vi "FT10_Fornax Mono1 Coag Power Down.vi"(11 "Message Handling Cluster in":T1={"Fornax Connected?"=refnum, "Unitherm Connected?"=refnum, "M4X Connected?"=refnum, "Unitherm Connect/Disconnect"=refnum, "Fornax Connection"=refnum, "UNITHERM Connection"="", "M4X Connection"=0, "FPGA VI Reference Out"=refnum, "PXI-7854R Connected?"=refnum, "Fornax Connect/Disconnect"=refnum, "7854 Connect/Disconnect"=refnum, "M4X Connect/Disconnect"=refnum, "Config cluster"={"Unitherm Port"="", "Simulate Values"=FALSE, "Fornax Connect Attempts"=0}, "Log Queue"=refnum, "Log Analysis Cluster - Current"={"RMS"=0.0, "Envelope Frequency"=0.0, "Peak"=0.0, "Crest Factor"=0.0, "Duty Cyle %"=0.0, "P-P"=0.0, "Frequency"=0.0, "THD"=0.0, "Postive Peak"=0.0, "Negative Peak"=0.0, "Mag_H1"=0.0, "Phase_H1"=0.0, "Mag_H3"=0.0, "Phase_H3"=0.0, "Mag_H5"=0.0, "Phase_H5"=0.0}, "Log Waveform Cluster - Current"={"t0"=timestamp(0 s since 1904-01-01), "dt"=1.0, "Y"=[]}, "Log Time"=timestamp(0 s since 1904-01-01), "Log Flag"=FALSE, "Log - Activation Settings Cluster"={"Log - Unitherm Load"="", "Log - Port"="", "Log - Mode"="", "Log - Power Level"=""}, "Log - Port Mode Cluster"={"Mono1 Cut Enum"=enum."Pure", "Mono2 Cut Enum"=enum."Pure", "Mono1 Coag Enum"=enum."Fulgerate", "Mono2 Coag Enum"=enum."Fulgerate", "Bipolar Enum"=enum."Standard"}, "Log Analysis Cluster - Diff Voltage"={"RMS"=0.0, "Envelope Frequency"=0.0, "Peak"=0.0, "Crest Factor"=0.0, "Duty Cyle %"=0.0, "P-P"=0.0, "Frequency"=0.0, "THD"=0.0, "Postive Peak"=0.0, "Negative Peak"=0.0, "Mag_H1"=0.0, "Phase_H1"=0.0, "Mag_H3"=0.0, "Phase_H3"=0.0, "Mag_H5"=0.0, "Phase_H5"=0.0}, "Log Waveform Cluster - Diff Voltage"={"t0"=timestamp(0 s since 1904-01-01), "dt"=1.0, "Y"=[]}, "Indicator Cluster"={"Mono1 - Cut Power"=refnum, "Mono1 - Coag Power"=refnum, "Mono2 - Cut Power"=refnum, "Mono2 - Coag Power"=refnum, "Bipolar Power"=refnum, "Mono1 Cut Enum"=refnum, "Mono1 Coag Enum"=refnum, "Mono2 Cut Enum"=refnum, "Mono2 Coag Enum"=refnum, "Bipolar Enum"=refnum}, "Log Power Level Cluster"={"Log Mono1 Cut Power"="", "Log Mono1 Coag Power"="", "Log Mono2 Cut Power"="", "Log Mono2 Coag Power"="", "Log Bipolar Power"=""}, "Footswitch Cluster"={"PXI-2565 reset device (boolean value)"=TRUE, "topology name"="2565/16-SPST", "PXI-2565 simulate (boolean value)"=FALSE, "PXI-2565 resource name"=""}}) -> (3 "Message Handling Cluster out":T1={"Fornax Connected?"=refnum, "Unitherm Connected?"=refnum, "M4X Connected?"=refnum, "Unitherm Connect/Disconnect"=refnum, "Fornax Connection"=refnum, "UNITHERM Connection"="", "M4X Connection"=0, "FPGA VI Reference Out"=refnum, "PXI-7854R Connected?"=refnum, "Fornax Connect/Disconnect"=refnum, "7854 Connect/Disconnect"=refnum, "M4X Connect/Disconnect"=refnum, "Config cluster"={"Unitherm Port"="", "Simulate Values"=FALSE, "Fornax Connect Attempts"=0}, "Log Queue"=refnum, "Log Analysis Cluster - Current"={"RMS"=0.0, "Envelope Frequency"=0.0, "Peak"=0.0, "Crest Factor"=0.0, "Duty Cyle %"=0.0, "P-P"=0.0, "Frequency"=0.0, "THD"=0.0, "Postive Peak"=0.0, "Negative Peak"=0.0, "Mag_H1"=0.0, "Phase_H1"=0.0, "Mag_H3"=0.0, "Phase_H3"=0.0, "Mag_H5"=0.0, "Phase_H5"=0.0}, "Log Waveform Cluster - Current"={"t0"=timestamp(0 s since 1904-01-01), "dt"=1.0, "Y"=[]}, "Log Time"=timestamp(0 s since 1904-01-01), "Log Flag"=FALSE, "Log - Activation Settings Cluster"={"Log - Unitherm Load"="", "Log - Port"="", "Log - Mode"="", "Log - Power Level"=""}, "Log - Port Mode Cluster"={"Mono1 Cut Enum"=enum."Pure", "Mono2 Cut Enum"=enum."Pure", "Mono1 Coag Enum"=enum."Fulgerate", "Mono2 Coag Enum"=enum."Fulgerate", "Bipolar Enum"=enum."Standard"}, "Log Analysis Cluster - Diff Voltage"={"RMS"=0.0, "Envelope Frequency"=0.0, "Peak"=0.0, "Crest Factor"=0.0, "Duty Cyle %"=0.0, "P-P"=0.0, "Frequency"=0.0, "THD"=0.0, "Postive Peak"=0.0, "Negative Peak"=0.0, "Mag_H1"=0.0, "Phase_H1"=0.0, "Mag_H3"=0.0, "Phase_H3"=0.0, "Mag_H5"=0.0, "Phase_H5"=0.0}, "Log Waveform Cluster - Diff Voltage"={"t0"=timestamp(0 s since 1904-01-01), "dt"=1.0, "Y"=[]}, "Indicator Cluster"={"Mono1 - Cut Power"=refnum, "Mono1 - Coag Power"=refnum, "Mono2 - Cut Power"=refnum, "Mono2 - Coag Power"=refnum, "Bipolar Power"=refnum, "Mono1 Cut Enum"=refnum, "Mono1 Coag Enum"=refnum, "Mono2 Cut Enum"=refnum, "Mono2 Coag Enum"=refnum, "Bipolar Enum"=refnum}, "Log Power Level Cluster"={"Log Mono1 Cut Power"="", "Log Mono1 Coag Power"="", "Log Mono2 Cut Power"="", "Log Mono2 Coag Power"="", "Log Bipolar Power"=""}, "Footswitch Cluster"={"PXI-2565 reset device (boolean value)"=TRUE, "topology name"="2565/16-SPST", "PXI-2565 simulate (boolean value)"=FALSE, "PXI-2565 resource name"=""}})   [LabVIEW 2024]
doc: "Decrease power level on Mono1 Coag"
uses:
  Controls/Control_Message Handling Cluster.ctl
  Controls/Control_M4X Connection.ctl
  Controls/Control_PXI-7854R FPGA Reference.ctl
  Controls/Control_Config Cluster.ctl
  Controls/Control_Config Unitherm Port.ctl
  Controls/Control_Config Simulate Values.ctl
  Controls/Control_Config Fornax Connect Attempts.ctl
  Controls/Control_Log Queue.ctl
  Controls/Control_Log Cluster.ctl
  Controls/Control_Log Time.ctl
  Controls/Control_Log Waveform Cluster - Current.ctl
  Controls/Control_Log Analysis Cluster - Current.ctl
  Controls/Control_Log Activation Settings Cluster.ctl
  Controls/Control_Log Unitherm Load.ctl
  Controls/Control_Log Port.ctl
  Controls/Control_Log Mode.ctl
  Controls/Control_Log Power Level.ctl
  Controls/Control_Log Waveform Cluster - Diff Voltage.ctl
  Controls/Control_Log Analysis Cluster - Diff Voltage.ctl
  Controls/Control_Log Flag.ctl
  Controls/Control_Log Port Mode Cluster.ctl
  Controls/Control_Fornax Mono1 Cut Enum.ctl
  Controls/Control_Fornax Mono2 Cut Enum.ctl
  Controls/Control_Fornax Mono1 Coag Enum.ctl
  Controls/Control_Fornax Mono2 Coag Enum.ctl
  Controls/Control_Fornax Bipolar Enum.ctl
  Controls/Control_Indicator Cluster.ctl
  Controls/Control_Log Power Level Cluster.ctl
  Controls/Control_Log Mono1 Cut Power.ctl
  Controls/Control_Log Mono1 Coag Power.ctl
  Controls/Control_Log Mono2 Cut Power.ctl
  Controls/Control_Log Mono2 Coag Power.ctl
  Controls/Control_Log Bipolar Power.ctl
  Controls/Control_Footswitch Reset Device Bool.ctl
  <instrlib>/niSwitch/niSwitch.llb/niSwitch Topologies.ctl
  Controls/Control_Footswitch Simulate Bool.ctl
  Controls/Control_Footswitch Resource Name.ctl
  Controls/Control_Fornax Generator.ctl
  Controls/Control_Fornax Energy Channel ID.ctl
  Controls/Control_Fornax Instrument Type.ctl
  Controls/Control_Fornax Parameter Type.ctl
  Controls/Control_Fornax Parameter Value.ctl
  Controls/Control_Fornax Energy Mode.ctl
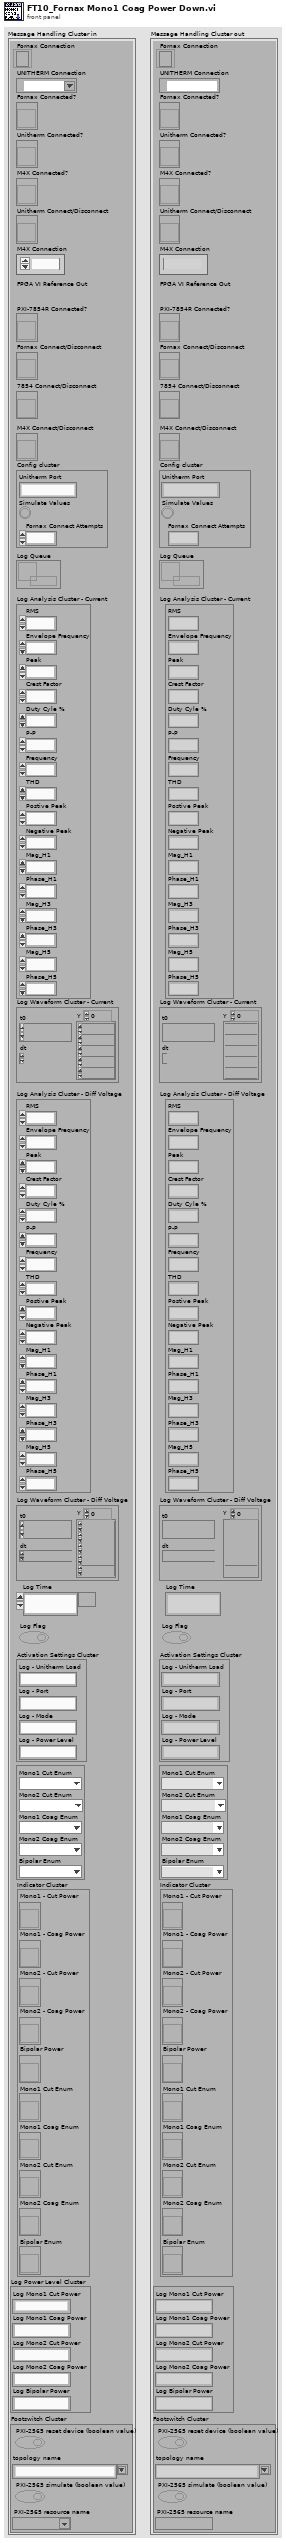
[diagram p1: front panel]
types:
  T1 = typedef "Control_Message Handling Cluster.ctl" = cluster{"Fornax Connected?":refnum<vi>, "Unitherm Connected?":refnum<vi>, "M4X Connected?":refnum<vi>, "Unitherm Connect/Disconnect":refnum<vi>, "Fornax Connection":refnum<k5>, "UNITHERM Connection":refnum<visa-resource-name>, "M4X Connection":T2, "FPGA VI Reference Out":T3, "PXI-7854R Connected?":refnum<vi>, "Fornax Connect/Disconnect":refnum<vi>, "7854 Connect/Disconnect":refnum<vi>, "M4X Connect/Disconnect":refnum<vi>, "Config cluster":T4, "Log Queue":T8, "Log Analysis Cluster - Current":T9, "Log Waveform Cluster - Current":T10, "Log Time":T11, "Log Flag":T12, "Log - Activation Settings Cluster":T13, "Log - Port Mode Cluster":T18, "Log Analysis Cluster - Diff Voltage":T24, "Log Waveform Cluster - Diff Voltage":T25, "Indicator Cluster":T26, "Log Power Level Cluster":T27, "Footswitch Cluster":cluster{"PXI-2565 reset device (boolean value)":T33, "topology name":T34, "PXI-2565 simulate (boolean value)":T35, "PXI-2565 resource name":T36}}
  T2 = typedef "Control_M4X Connection.ctl" = u32
  T3 = typedef "Control_PXI-7854R FPGA Reference.ctl" = refnum<k20>
  T4 = typedef "Control_Config Cluster.ctl" = cluster{"Unitherm Port":T5, "Simulate Values":T6, "Fornax Connect Attempts":T7}
  T5 = typedef "Control_Config Unitherm Port.ctl" = string
  T6 = typedef "Control_Config Simulate Values.ctl" = bool
  T7 = typedef "Control_Config Fornax Connect Attempts.ctl" = i32
  T8 = typedef "Control_Log Queue.ctl" = refnum<queue>
  T9 = typedef "Control_Log Analysis Cluster - Current.ctl" = cluster{"RMS":dbl, "Envelope Frequency":dbl, "Peak":dbl, "Crest Factor":dbl, "Duty Cyle %":dbl, "P-P":dbl, "Frequency":dbl, "THD":dbl, "Postive Peak":dbl, "Negative Peak":dbl, "Mag_H1":dbl, "Phase_H1":dbl, "Mag_H3":dbl, "Phase_H3":dbl, "Mag_H5":dbl, "Phase_H5":dbl}
  T10 = typedef "Control_Log Waveform Cluster - Current.ctl" = waveform(dbl)
  T11 = typedef "Control_Log Time.ctl" = timestamp
  T12 = typedef "Control_Log Flag.ctl" = bool
  T13 = typedef "Control_Log Activation Settings Cluster.ctl" = cluster{"Log - Unitherm Load":T14, "Log - Port":T15, "Log - Mode":T16, "Log - Power Level":T17}
  T14 = typedef "Control_Log Unitherm Load.ctl" = string
  T15 = typedef "Control_Log Port.ctl" = string
  T16 = typedef "Control_Log Mode.ctl" = string
  T17 = typedef "Control_Log Power Level.ctl" = string
  T18 = typedef "Control_Log Port Mode Cluster.ctl" = cluster{"Mono1 Cut Enum":T19, "Mono2 Cut Enum":T20, "Mono1 Coag Enum":T21, "Mono2 Coag Enum":T22, "Bipolar Enum":T23}
  T19 = typedef "Control_Fornax Mono1 Cut Enum.ctl" = enum16{"Pure", "Blend"}
  T20 = typedef "Control_Fornax Mono2 Cut Enum.ctl" = enum16{"Pure", "Blend"}
  T21 = typedef "Control_Fornax Mono1 Coag Enum.ctl" = enum16{"Fulgerate", "Spray"}
  T22 = typedef "Control_Fornax Mono2 Coag Enum.ctl" = enum16{"Fulgerate", "Spray"}
  T23 = typedef "Control_Fornax Bipolar Enum.ctl" = enum16{"Standard", "Macro", "Precision"}
  T24 = typedef "Control_Log Analysis Cluster - Diff Voltage.ctl" = cluster{"RMS":dbl, "Envelope Frequency":dbl, "Peak":dbl, "Crest Factor":dbl, "Duty Cyle %":dbl, "P-P":dbl, "Frequency":dbl, "THD":dbl, "Postive Peak":dbl, "Negative Peak":dbl, "Mag_H1":dbl, "Phase_H1":dbl, "Mag_H3":dbl, "Phase_H3":dbl, "Mag_H5":dbl, "Phase_H5":dbl}
  T25 = typedef "Control_Log Waveform Cluster - Diff Voltage.ctl" = waveform(dbl)
  T26 = typedef "Control_Indicator Cluster.ctl" = cluster{"Mono1 - Cut Power":refnum<vi>, "Mono1 - Coag Power":refnum<vi>, "Mono2 - Cut Power":refnum<vi>, "Mono2 - Coag Power":refnum<vi>, "Bipolar Power":refnum<vi>, "Mono1 Cut Enum":refnum<vi>, "Mono1 Coag Enum":refnum<vi>, "Mono2 Cut Enum":refnum<vi>, "Mono2 Coag Enum":refnum<vi>, "Bipolar Enum":refnum<vi>}
  T27 = typedef "Control_Log Power Level Cluster.ctl" = cluster{"Log Mono1 Cut Power":T28, "Log Mono1 Coag Power":T29, "Log Mono2 Cut Power":T30, "Log Mono2 Coag Power":T31, "Log Bipolar Power":T32}
  T28 = typedef "Control_Log Mono1 Cut Power.ctl" = string
  T29 = typedef "Control_Log Mono1 Coag Power.ctl" = string
  T30 = typedef "Control_Log Mono2 Cut Power.ctl" = string
  T31 = typedef "Control_Log Mono2 Coag Power.ctl" = string
  T32 = typedef "Control_Log Bipolar Power.ctl" = string
  T33 = typedef "Control_Footswitch Reset Device Bool.ctl" = bool
  T34 = typedef "niSwitch Topologies.ctl" = string
  T35 = typedef "Control_Footswitch Simulate Bool.ctl" = bool
  T36 = typedef "Control_Footswitch Resource Name.ctl" = refnum<k15>
  T37 = typedef "Control_Fornax Energy Mode.ctl" = enum16{"SPRAY_MODE", "CUT_MODE", "BLEND_MODE", "FULGERATE_MODE", "BIPOLAR_MODE", "VESSEL_SEALING_MODE", "VALLEYLAB_MODE", "BIPOLAR_RESECTION_CUT_MODE", "BIPOLAR_RESECTION_COAG_MODE", "AUTOBIPOLAR_MODE", "VIPER_HLA", "SOFT_COAG_MODE", "ECUT_MODE", "SHARED_SPRAY_MODE", "SHARED_FULGERATE_MODE", "CARDIO_MONO_MODE", "CARDIO_BIPOLAR_MODE", "BIPOLAR_LOW_MODE", "BIPOLAR_MACRO_MODE", "BIPOLAR_STANDARD_MODE", "BIPOLAR_MEDIUM_MODE", "VL_ENDOSCOPY_MODE", "NUM_ENERGY_MODES"}
  T38 = typedef "Control_Fornax Parameter Value.ctl" = i32
  T39 = typedef "Control_Fornax Parameter Type.ctl" = enum16{"POWER_PARAMETER", "CUT_MODALITY_POWER_PARAMETER", "COAG_MODALITY_POWER_PARAMETER", "VL_MODALITY_POWER_PARAMETER", "BY_MODE_POWER_PARAMETER", "VL_ENDO_CUT_MODALITY_POWER_PARAMETER", "VL_ENDO_COAG_MODALITY_POWER_PARAMETER", "VL_ENDO_COAG_ON_CUT_MODALITY_POWER_PARAMETER", "MODE_PARAMETER   (for changing Bipolar mode)", "CUT_MODALITY_MODE_PARAMETER  (for changing monopolar cut mode)", "COAG_MODALITY_MODE_PARAMETER (for changing monopolar coag mode)", "VL_ENDO_COAG_MODALITY_MODE_PARAMETER", "VL_ENDO_CUT_INTERVAL_PARAMETER", "VL_ENDO_CUT_DURATION_PARAMETER", "POWER_BAR_PARAMETER", "MAX_ACTIVATION_MSEC_TIME_PARAMETER", "AUTOBIPOLAR_DELAY_MSEC_TIME", "VL_ENDO_COAG_QUICK_ACCESS_PARAMETER"}
  T40 = typedef "Control_Fornax Instrument Type.ctl" = enum16{"INSTRUMENT_TYPE_UNKNOWN", "INSTRUMENT_TYPE_MONOPOLAR", "INSTRUMENT_TYPE_BIPOLAR", "INSTRUMENT_TYPE_TRIVERSE", "INSTRUMENT_TYPE_LIGASURE", "INSTRUMENT_TYPE_ADVANCE_II", "INSTRUMENT_TYPE_BIPOLAR_RESECTION", "INSTRUMENT_TYPE_HOOK", "INSTRUMENT_TYPE_BIZACT", "INSTRUMENT_TYPE_CARDIOBLATE_BIP", "INSTRUMENT_TYPE_CARDIOBLATE_BIP_GEMINI_S", "INSTRUMENT_TYPE_CARDIOBLATE_MONO", "INSTRUMENT_TYPE_ULTRASONIC", "INSTRUMENT_TYPE_MONOPOLAR_GI ", "INSTRUMENT_TYPE_GOLDILOCKS "}
  T41 = typedef "Control_Fornax Energy Channel ID.ctl" = enum16{"EC_MONO_1  ", "EC_BIPOLAR  ", "EC_MONO_2  ", "EC_ADVANCED  ", "EC_ADVANCED_ECUT  ", "EC_ADVANCED_DCUT  ", "EC_SHARED_COAG  ", "EC_INTERNAL_BIP_CAL  "}
  T42 = typedef "Control_Fornax Generator.ctl" = string
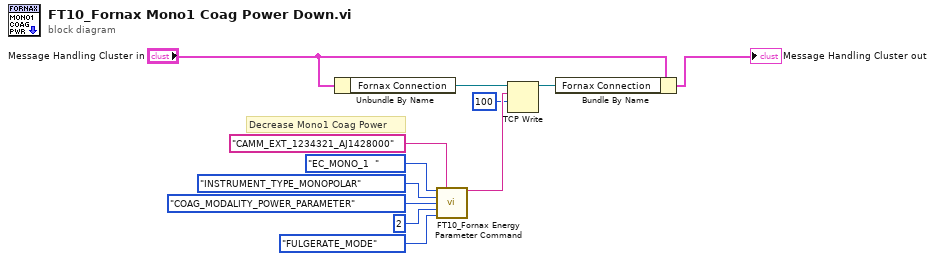
[diagram p0: block diagram]
diagram:
  # "Decrease Mono1 Coag Power"
  n1 = Unbundle By Name("Message Handling Cluster in") -> ("Fornax Connection"=w3:refnum<k5>)
  n2 = call "FT10_Fornax Energy Parameter Command.vi"("Energy Channel ID"=Control_Fornax_Energy_Channel_ID."EC_MONO_1  ", "Generator"=T42 "CAMM_EXT_1234321_AJ1428000", "Instrument Type"=Control_Fornax_Instrument_Type."INSTRUMENT_TYPE_MONOPOLAR", "Parameter Type"=Control_Fornax_Parameter_Type."COAG_MODALITY_POWER_PARAMETER", "Parameter Value"=T38 2, "Energy Mode"=Control_Fornax_Energy_Mode."FULGERATE_MODE") -> ("JSON Command"=w11:string)  [unwired: 9 in]
  n3 = TCP Write(connection ID=w3, data in=w11, 9:100 ("timeout ms (25000)")) -> (connection ID out=w4:refnum<k5>)  [unwired: 1 in, 2 out]
  n4 = Bundle By Name(cluster="Message Handling Cluster in", "Fornax Connection"=w4) -> (→"Message Handling Cluster out":T1)
